vi "Export Error.vi"(6 "Stack Trace":string, 8 "error in (no error)":errorcluster, 9 "Type":string, 10 "Message":string, 11 "Node in":refnum<k20>) -> (0 "error out":errorcluster, 3 "Node out":refnum<k20>)   [LabVIEW 2013, in "JUnit for Azure Pipelines.lvclass"]
uses:
  JUnit for Azure Pipelines.lvclass
  <vilib>/xml/Close Reference(Node).vi
  <vilib>/xml/NI_XML.lvlib
  XML/XML.lvlib
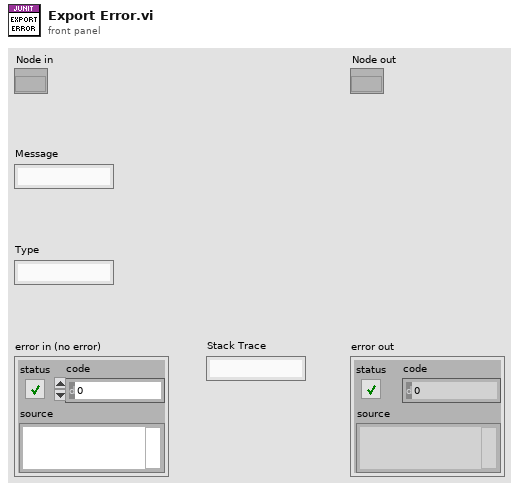
[diagram p1: front panel]
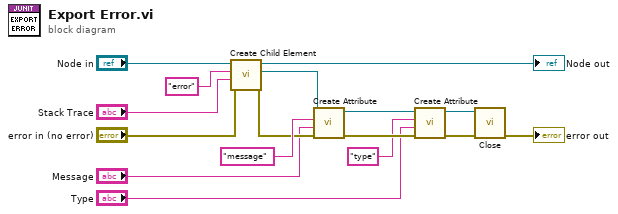
[diagram p0: block diagram]
diagram:
  n1 = call "Create Child Element.vi"("error in (no error)"="error in (no error)", "Value (\"\")"="Stack Trace", "Name"="error" ("Tag Name"), "Element in"="Node in") -> ("error out"=w6:errorcluster, "Child Element"=w7:refnum<k20>, "Element out"=→"Node out":refnum<k20>)  [unwired: 5 in]
  n2 = call "Create Attribute.vi"("error in (no error)"=w6, "Value"="Message", "Name"="message" ("Attribute Name"), "Element in"=w7) -> ("error out"=w9:errorcluster, "Element out"=w10:refnum<k20>)  [unwired: 6 in]
  n3 = call "Create Attribute.vi"("error in (no error)"=w9, "Value"="Type", "Name"="type" ("Attribute Name"), "Element in"=w10) -> ("error out"=w4:errorcluster, "Element out"=w5:refnum<k20>)  [unwired: 6 in]
  n4 = call-poly <vilib>:"Close.vi"("error in (no error)"=w4, "node"=w5) -> ("error out"=→"error out":errorcluster)  [unwired: 7 in]
